vi "Exponential Test.vi"() -> ()   [LabVIEW 2014]
uses:
  <vilib>/Math Plots/3D Math Plots/3D Scatter/3D Scatter XCtrl/3D Scatter.xctl
  <vilib>/Math Plots/3D Math Plots/3D Scatter/3D Scatter Datatype/Public/Plot Helper (Vector).vi
  <vilib>/Analysis/1siggen.llb/Ramp Pattern by Delta.vi
  Math Utilities.lvlib
  <vilib>/Analysis/NI_AALBase.lvlib
  <vilib>/measure/NI_MABase.lvlib
  <vilib>/Math Plots/3D Math Plots/3D Scatter/3D Scatter Datatype/3D Scatter Datatype.lvclass
panel:
  out "Selected Noise Level":dbl
  in  "noise index":i32
  out "etau'":cluster{dbl[], dbl[]}[](graph)=[{[0.0, 0.05, 0.1, 0.15, 0.2, 0.25, 0.3, 0.35, 0.4, 0.45, 0.5, 0.55, 0.6, 0.65, 0.7, 0.75, 0.8, 0.85, 0.9, 0.95, 1.0, 1.05, 1.1, 1.15, 1.2, 1.25, 1.3, 1.35, 1.4, 1.45, 1.5, 1.55, 1.6, 1.65, 1.7, 1.75, 1.8, 1.85, 1.9, 1.95, 2.0, 2.05, 2.1, 2.15, 2.2, 2.25, 2.3, 2.35, 2.4, 2.45, 2.5, 2.55, 2.6, 2.65, 2.7, 2.75, 2.8, 2.85, 2.9, 2.95, 3.0, 3.05, 3.1, 3.15, 3.2, 3.25, 3.3, 3.35, 3.4, 3.45, 3.5, 3.55, 3.6, 3.65, 3.7, 3.75, 3.8, 3.85, 3.9, 3.95, 4.0, 4.05, 4.1, 4.15, 4.2, 4.25, 4.3, 4.35, 4.4, 4.45, 4.5, 4.55, 4.6, 4.65, 4.7, 4.75, 4.8, 4.85, 4.9, 4.95], [0.960541444934628, 1.0300287046137588, 0.8896412059372913, 0.8809320306793802, 0.7883247330312061, 0.8176833763391205, 0.6447128922258879, 0.6273332809368509, 0.6605682518837364, 0.6670014264280115, 0.583805564940926, 0.675732358744051, 0.4639846933111526, 0.6202542521121932, 0.5597277145279371, 0.5135564243561868, 0.5062733727780937, 0.3613578160271843, 0.4475233678516537, 0.3793968608808492, 0.43724877411342006, 0.3597384315625127, 0.2373620816547545, 0.22453592933762084, 0.29842459974751334, 0.3050071640074105, 0.2359236866011837, 0.24302284161365773, 0.23920428907537397, 0.2700720254736181, 0.1918881215092269, 0.2316375620963971, 0.2698374059004593, 0.10938565371609907, 0.18228368619733432, 0.1995904055680095, 0.10262683454287629, 0.12951323626014882, 0.1883316121198414, 0.051005880662942066, 0.1882658145929273, 0.2253474344702741, 0.1072676376138868, 0.05420331503554107, 0.07073686122149538, 0.19072834912888081, 0.06489404614590896, 0.02340665923857653, 0.080727031502262, 0.053160478621205834, 0.1150566849039812, 0.08647339206694683, 0.17225004999139676, 0.14385515421965545, 0.09476811084635094, 0.08535850566392958, 0.042453337460426295, -0.005111835078437502, 0.1266720101202937, 0.08798857698089546, 0.06448330591172151, 0.012535109492323698, -0.02180050629331399, 0.13921091410606592, -0.00448119475112807, 0.025953771409014427, 0.09196924940378937, 0.1251848736523793, 0.09872337746996236, -0.02796928416987523, -0.0439093646999277, 0.07577564143222511, -0.03469012345164275, 0.1000290582787502, 0.07570130581455305, 0.10981843839037647, 0.030883562880611268, 0.05482327411195698, -0.016277970417741722, 0.0739773731669493, 0.11823230258380474, 0.022378034520468177, 0.015118202748243353, 0.06436576688809863, 0.034369714129696256, -0.07590989562072355, 0.11223730777048424, -0.05352288298618646, 0.059251144916092124, -0.054463595365239675, 0.10903521158421503, 0.07349724843361212, -0.04763649889666532, 0.05840026342982382, -0.06312941047179772, -0.04841695002411584, 0.0871009289199655, -0.08241366972549377, 0.06657825659960447, 0.01870496404000565]}, {[0.0, 0.1, 0.2, 0.3, 0.4, 0.5, 0.6, 0.7, 0.8, 0.9, 1.0, 1.1, 1.2, 1.3, 1.4, 1.5, 1.6, 1.7, 1.8, 1.9, 2.0, 2.1, 2.2, 2.3, 2.4, 2.5, 2.6, 2.7, 2.8, 2.9, 3.0, 3.1, 3.2, 3.3, 3.4, 3.5, 3.6, 3.7, 3.8, 3.9, 4.0, 4.1, 4.2, 4.3, 4.4, 4.5, 4.6, 4.7, 4.8, 4.9], [1.0489118049155677, 0.9828657414468108, 0.7287092685494896, 0.7402604459878791, 0.5870346294794287, 0.586721816909444, 0.45440624030548527, 0.5237279303930864, 0.3972561140761981, 0.33254829917367884, 0.34818621735970484, 0.3989198005547301, 0.34947614865970883, 0.20883760536624074, 0.20965525245589398, 0.26857776347019313, 0.23122560558625996, 0.23874984457269088, 0.15561255360224382, 0.1418318343504817, 0.11626272362059906, 0.16392580193843515, 0.033834333279495796, 0.0778706880250746, -0.007929789367372514, 0.005419938340864641, 0.04836411782582296, 0.12887685022889384, 0.15987281329989583, 0.002826123372845442, 0.044361005460079386, 0.01107762227846102, 0.027130325332161268, -0.0329011607483985, -0.00976715691082395, -0.01851382955827155, -0.02912386416561294, 0.05216385233514075, -0.01890067181650635, -0.06324219670124576, -0.06851294508129749, -0.002777132357630538, -0.014512361417010615, 0.08683899542703284, 0.08258002031887463, -0.024344103284262092, 0.0437718075673618, -0.06155030056137617, 0.06644365751447188, 0.05045892575985402]}, {[0.0, 0.2, 0.4, 0.6, 0.8, 1.0, 1.2, 1.4, 1.6, 1.8, 2.0, 2.2, 2.4, 2.6, 2.8, 3.0, 3.2, 3.4, 3.6, 3.8, 4.0, 4.2, 4.4, 4.6, 4.8], [1.0166445888668472, 0.8965127205564365, 0.6746646020918559, 0.5979355379266843, 0.4854152133224972, 0.3872720439703156, 0.3657660253817956, 0.30351089738058307, 0.2198216708301479, 0.20705366479755255, 0.06903085210606028, 0.16530276730729707, 0.15939586940300982, 0.083518667159258, 0.0640925481270926, 0.06369433525293566, 0.04352509905837727, 0.036281546977637566, 0.043303657543107665, 0.08611682194308087, 0.029590496545093097, -0.01733169050921223, -0.024397551503856203, -0.05234666017391198, -0.03711380387257694]}, {[0.0, 0.5, 1.0, 1.5, 2.0, 2.5, 3.0, 3.5, 4.0, 4.5], [1.0623034361710997, 0.5317673867138099, 0.42771698929286195, 0.17661929472640508, 0.05033997654512429, 0.03973823954012479, 0.09664850852882598, 0.07924682307796599, 0.11213514888422532, 0.10083456799625037]}, {[0.0, 1.0, 2.0, 3.0, 4.0], [1.097092230716005, 0.32607780199041114, 0.13609726715261378, 0.0013463089040823967, 0.0574822313090591]}]
  out "tau'":cluster{dbl[], dbl[]}[](graph)=[{[0.0, 0.05, 0.1, 0.15, 0.2, 0.25, 0.3, 0.35, 0.4, 0.45, 0.5, 0.55, 0.6, 0.65, 0.7, 0.75, 0.8, 0.85, 0.9, 0.95, 1.0, 1.05, 1.1, 1.15, 1.2, 1.25, 1.3, 1.35, 1.4, 1.45, 1.5, 1.55, 1.6, 1.65, 1.7, 1.75, 1.8, 1.85, 1.9, 1.95, 2.0, 2.05, 2.1, 2.15, 2.2, 2.25, 2.3, 2.35, 2.4, 2.45, 2.5, 2.55, 2.6, 2.65, 2.7, 2.75, 2.8, 2.85, 2.9, 2.95, 3.0, 3.05, 3.1, 3.15, 3.2, 3.25, 3.3, 3.35, 3.4, 3.45, 3.5, 3.55, 3.6, 3.65, 3.7, 3.75, 3.8, 3.85, 3.9, 3.95, 4.0, 4.05, 4.1, 4.15, 4.2, 4.25, 4.3, 4.35, 4.4, 4.45, 4.5, 4.55, 4.6, 4.65, 4.7, 4.75, 4.8, 4.85, 4.9, 4.95], [0.960541444934628, 1.0300287046137588, 0.8896412059372913, 0.8809320306793802, 0.7883247330312061, 0.8176833763391205, 0.6447128922258879, 0.6273332809368509, 0.6605682518837364, 0.6670014264280115, 0.583805564940926, 0.675732358744051, 0.4639846933111526, 0.6202542521121932, 0.5597277145279371, 0.5135564243561868, 0.5062733727780937, 0.3613578160271843, 0.4475233678516537, 0.3793968608808492, 0.43724877411342006, 0.3597384315625127, 0.2373620816547545, 0.22453592933762084, 0.29842459974751334, 0.3050071640074105, 0.2359236866011837, 0.24302284161365773, 0.23920428907537397, 0.2700720254736181, 0.1918881215092269, 0.2316375620963971, 0.2698374059004593, 0.10938565371609907, 0.18228368619733432, 0.1995904055680095, 0.10262683454287629, 0.12951323626014882, 0.1883316121198414, 0.051005880662942066, 0.1882658145929273, 0.2253474344702741, 0.1072676376138868, 0.05420331503554107, 0.07073686122149538, 0.19072834912888081, 0.06489404614590896, 0.02340665923857653, 0.080727031502262, 0.053160478621205834, 0.1150566849039812, 0.08647339206694683, 0.17225004999139676, 0.14385515421965545, 0.09476811084635094, 0.08535850566392958, 0.042453337460426295, -0.005111835078437502, 0.1266720101202937, 0.08798857698089546, 0.06448330591172151, 0.012535109492323698, -0.02180050629331399, 0.13921091410606592, -0.00448119475112807, 0.025953771409014427, 0.09196924940378937, 0.1251848736523793, 0.09872337746996236, -0.02796928416987523, -0.0439093646999277, 0.07577564143222511, -0.03469012345164275, 0.1000290582787502, 0.07570130581455305, 0.10981843839037647, 0.030883562880611268, 0.05482327411195698, -0.016277970417741722, 0.0739773731669493, 0.11823230258380474, 0.022378034520468177, 0.015118202748243353, 0.06436576688809863, 0.034369714129696256, -0.07590989562072355, 0.11223730777048424, -0.05352288298618646, 0.059251144916092124, -0.054463595365239675, 0.10903521158421503, 0.07349724843361212, -0.04763649889666532, 0.05840026342982382, -0.06312941047179772, -0.04841695002411584, 0.0871009289199655, -0.08241366972549377, 0.06657825659960447, 0.01870496404000565]}, {[0.0, 0.1, 0.2, 0.3, 0.4, 0.5, 0.6, 0.7, 0.8, 0.9, 1.0, 1.1, 1.2, 1.3, 1.4, 1.5, 1.6, 1.7, 1.8, 1.9, 2.0, 2.1, 2.2, 2.3, 2.4, 2.5, 2.6, 2.7, 2.8, 2.9, 3.0, 3.1, 3.2, 3.3, 3.4, 3.5, 3.6, 3.7, 3.8, 3.9, 4.0, 4.1, 4.2, 4.3, 4.4, 4.5, 4.6, 4.7, 4.8, 4.9], [1.0489118049155677, 0.9828657414468108, 0.7287092685494896, 0.7402604459878791, 0.5870346294794287, 0.586721816909444, 0.45440624030548527, 0.5237279303930864, 0.3972561140761981, 0.33254829917367884, 0.34818621735970484, 0.3989198005547301, 0.34947614865970883, 0.20883760536624074, 0.20965525245589398, 0.26857776347019313, 0.23122560558625996, 0.23874984457269088, 0.15561255360224382, 0.1418318343504817, 0.11626272362059906, 0.16392580193843515, 0.033834333279495796, 0.0778706880250746, -0.007929789367372514, 0.005419938340864641, 0.04836411782582296, 0.12887685022889384, 0.15987281329989583, 0.002826123372845442, 0.044361005460079386, 0.01107762227846102, 0.027130325332161268, -0.0329011607483985, -0.00976715691082395, -0.01851382955827155, -0.02912386416561294, 0.05216385233514075, -0.01890067181650635, -0.06324219670124576, -0.06851294508129749, -0.002777132357630538, -0.014512361417010615, 0.08683899542703284, 0.08258002031887463, -0.024344103284262092, 0.0437718075673618, -0.06155030056137617, 0.06644365751447188, 0.05045892575985402]}, {[0.0, 0.2, 0.4, 0.6, 0.8, 1.0, 1.2, 1.4, 1.6, 1.8, 2.0, 2.2, 2.4, 2.6, 2.8, 3.0, 3.2, 3.4, 3.6, 3.8, 4.0, 4.2, 4.4, 4.6, 4.8], [1.0166445888668472, 0.8965127205564365, 0.6746646020918559, 0.5979355379266843, 0.4854152133224972, 0.3872720439703156, 0.3657660253817956, 0.30351089738058307, 0.2198216708301479, 0.20705366479755255, 0.06903085210606028, 0.16530276730729707, 0.15939586940300982, 0.083518667159258, 0.0640925481270926, 0.06369433525293566, 0.04352509905837727, 0.036281546977637566, 0.043303657543107665, 0.08611682194308087, 0.029590496545093097, -0.01733169050921223, -0.024397551503856203, -0.05234666017391198, -0.03711380387257694]}, {[0.0, 0.5, 1.0, 1.5, 2.0, 2.5, 3.0, 3.5, 4.0, 4.5], [1.0623034361710997, 0.5317673867138099, 0.42771698929286195, 0.17661929472640508, 0.05033997654512429, 0.03973823954012479, 0.09664850852882598, 0.07924682307796599, 0.11213514888422532, 0.10083456799625037]}, {[0.0, 1.0, 2.0, 3.0, 4.0], [1.097092230716005, 0.32607780199041114, 0.13609726715261378, 0.0013463089040823967, 0.0574822313090591]}]
  out "output array":dbl[](array[numeric])
  out "Array 3":dbl[](array[numeric])
  out "Array 2":dbl[](array[numeric])
  in  "tau index":i32
  out "3D Scatter":refnum<class "3D Plot Datatype.lvclass">[](xcontrol)
  out "Array":T1(array[cluster])
  in  "taus (us)":dbl[](array[numeric])=[0.5, 1.0, 2.0, 5.0, 10.0, 20.0, 50.0, 100.0, 150.0]
  in  "Noise Levels":dbl[](array[numeric])=[0.0, 0.01, 0.05, 0.1, 0.2, 0.3, 0.4, 0.5, 1.0]
  in  "# Taus":dbl=5.0
  in  "Number of Samples":dbl=4000.0
  out "Taus":T2(graph)=[{"Sampling Frequencies (MHz)"=[20.0, 10.0, 5.0, 2.0, 1.0], [0.9656086307823587, 0.9866685202887719, 1.1569644501410312, 0.7662051282812012, 0.8285928880796682]}, {"Sampling Frequencies (MHz)"=[20.0, 10.0, 5.0, 2.0, 1.0], [0.026104009183676023, 0.034896410998791996, 0.03328061139393245, 0.07782595805221088, 0.07635392209771198]}, {"Sampling Frequencies (MHz)"=[20.0, 10.0, 5.0, 2.0, 1.0], [0.9408079235146063, 0.9408079235146063, 0.9408079235146063, 0.9408079235146063, 0.9408079235146063]}]
  out "Exponential":cluster{dbl[], dbl[]}[](graph)=[{[0.0, 0.05, 0.1, 0.15, 0.2, 0.25, 0.3, 0.35, 0.4, 0.45, 0.5, 0.55, 0.6, 0.65, 0.7, 0.75, 0.8, 0.85, 0.9, 0.95, 1.0, 1.05, 1.1, 1.15, 1.2, 1.25, 1.3, 1.35, 1.4, 1.45, 1.5, 1.55, 1.6, 1.65, 1.7, 1.75, 1.8, 1.85, 1.9, 1.95, 2.0, 2.05, 2.1, 2.15, 2.2, 2.25, 2.3, 2.35, 2.4, 2.45, 2.5, 2.55, 2.6, 2.65, 2.7, 2.75, 2.8, 2.85, 2.9, 2.95, 3.0, 3.05, 3.1, 3.15, 3.2, 3.25, 3.3, 3.35, 3.4, 3.45, 3.5, 3.55, 3.6, 3.65, 3.7, 3.75, 3.8, 3.85, 3.9, 3.95, 4.0, 4.05, 4.1, 4.15, 4.2, 4.25, 4.3, 4.35, 4.4, 4.45, 4.5, 4.55, 4.6, 4.65, 4.7, 4.75, 4.8, 4.85, 4.9, 4.95], [0.960541444934628, 1.0300287046137588, 0.8896412059372913, 0.8809320306793802, 0.7883247330312061, 0.8176833763391205, 0.6447128922258879, 0.6273332809368509, 0.6605682518837364, 0.6670014264280115, 0.583805564940926, 0.675732358744051, 0.4639846933111526, 0.6202542521121932, 0.5597277145279371, 0.5135564243561868, 0.5062733727780937, 0.3613578160271843, 0.4475233678516537, 0.3793968608808492, 0.43724877411342006, 0.3597384315625127, 0.2373620816547545, 0.22453592933762084, 0.29842459974751334, 0.3050071640074105, 0.2359236866011837, 0.24302284161365773, 0.23920428907537397, 0.2700720254736181, 0.1918881215092269, 0.2316375620963971, 0.2698374059004593, 0.10938565371609907, 0.18228368619733432, 0.1995904055680095, 0.10262683454287629, 0.12951323626014882, 0.1883316121198414, 0.051005880662942066, 0.1882658145929273, 0.2253474344702741, 0.1072676376138868, 0.05420331503554107, 0.07073686122149538, 0.19072834912888081, 0.06489404614590896, 0.02340665923857653, 0.080727031502262, 0.053160478621205834, 0.1150566849039812, 0.08647339206694683, 0.17225004999139676, 0.14385515421965545, 0.09476811084635094, 0.08535850566392958, 0.042453337460426295, -0.005111835078437502, 0.1266720101202937, 0.08798857698089546, 0.06448330591172151, 0.012535109492323698, -0.02180050629331399, 0.13921091410606592, -0.00448119475112807, 0.025953771409014427, 0.09196924940378937, 0.1251848736523793, 0.09872337746996236, -0.02796928416987523, -0.0439093646999277, 0.07577564143222511, -0.03469012345164275, 0.1000290582787502, 0.07570130581455305, 0.10981843839037647, 0.030883562880611268, 0.05482327411195698, -0.016277970417741722, 0.0739773731669493, 0.11823230258380474, 0.022378034520468177, 0.015118202748243353, 0.06436576688809863, 0.034369714129696256, -0.07590989562072355, 0.11223730777048424, -0.05352288298618646, 0.059251144916092124, -0.054463595365239675, 0.10903521158421503, 0.07349724843361212, -0.04763649889666532, 0.05840026342982382, -0.06312941047179772, -0.04841695002411584, 0.0871009289199655, -0.08241366972549377, 0.06657825659960447, 0.01870496404000565]}, {[0.0, 0.1, 0.2, 0.3, 0.4, 0.5, 0.6, 0.7, 0.8, 0.9, 1.0, 1.1, 1.2, 1.3, 1.4, 1.5, 1.6, 1.7, 1.8, 1.9, 2.0, 2.1, 2.2, 2.3, 2.4, 2.5, 2.6, 2.7, 2.8, 2.9, 3.0, 3.1, 3.2, 3.3, 3.4, 3.5, 3.6, 3.7, 3.8, 3.9, 4.0, 4.1, 4.2, 4.3, 4.4, 4.5, 4.6, 4.7, 4.8, 4.9], [1.0489118049155677, 0.9828657414468108, 0.7287092685494896, 0.7402604459878791, 0.5870346294794287, 0.586721816909444, 0.45440624030548527, 0.5237279303930864, 0.3972561140761981, 0.33254829917367884, 0.34818621735970484, 0.3989198005547301, 0.34947614865970883, 0.20883760536624074, 0.20965525245589398, 0.26857776347019313, 0.23122560558625996, 0.23874984457269088, 0.15561255360224382, 0.1418318343504817, 0.11626272362059906, 0.16392580193843515, 0.033834333279495796, 0.0778706880250746, -0.007929789367372514, 0.005419938340864641, 0.04836411782582296, 0.12887685022889384, 0.15987281329989583, 0.002826123372845442, 0.044361005460079386, 0.01107762227846102, 0.027130325332161268, -0.0329011607483985, -0.00976715691082395, -0.01851382955827155, -0.02912386416561294, 0.05216385233514075, -0.01890067181650635, -0.06324219670124576, -0.06851294508129749, -0.002777132357630538, -0.014512361417010615, 0.08683899542703284, 0.08258002031887463, -0.024344103284262092, 0.0437718075673618, -0.06155030056137617, 0.06644365751447188, 0.05045892575985402]}, {[0.0, 0.2, 0.4, 0.6, 0.8, 1.0, 1.2, 1.4, 1.6, 1.8, 2.0, 2.2, 2.4, 2.6, 2.8, 3.0, 3.2, 3.4, 3.6, 3.8, 4.0, 4.2, 4.4, 4.6, 4.8], [1.0166445888668472, 0.8965127205564365, 0.6746646020918559, 0.5979355379266843, 0.4854152133224972, 0.3872720439703156, 0.3657660253817956, 0.30351089738058307, 0.2198216708301479, 0.20705366479755255, 0.06903085210606028, 0.16530276730729707, 0.15939586940300982, 0.083518667159258, 0.0640925481270926, 0.06369433525293566, 0.04352509905837727, 0.036281546977637566, 0.043303657543107665, 0.08611682194308087, 0.029590496545093097, -0.01733169050921223, -0.024397551503856203, -0.05234666017391198, -0.03711380387257694]}, {[0.0, 0.5, 1.0, 1.5, 2.0, 2.5, 3.0, 3.5, 4.0, 4.5], [1.0623034361710997, 0.5317673867138099, 0.42771698929286195, 0.17661929472640508, 0.05033997654512429, 0.03973823954012479, 0.09664850852882598, 0.07924682307796599, 0.11213514888422532, 0.10083456799625037]}, {[0.0, 1.0, 2.0, 3.0, 4.0], [1.097092230716005, 0.32607780199041114, 0.13609726715261378, 0.0013463089040823967, 0.0574822313090591]}]
  in  "Run Calc":bool=TRUE
  in  "B":dbl
  in  "A":dbl=1.0
  in  "Sampling Frequencies (MHz)":dbl[](array[numeric])=[20.0, 15.0, 10.0, 8.0, 6.0, 5.0, 2.5, 1.0]
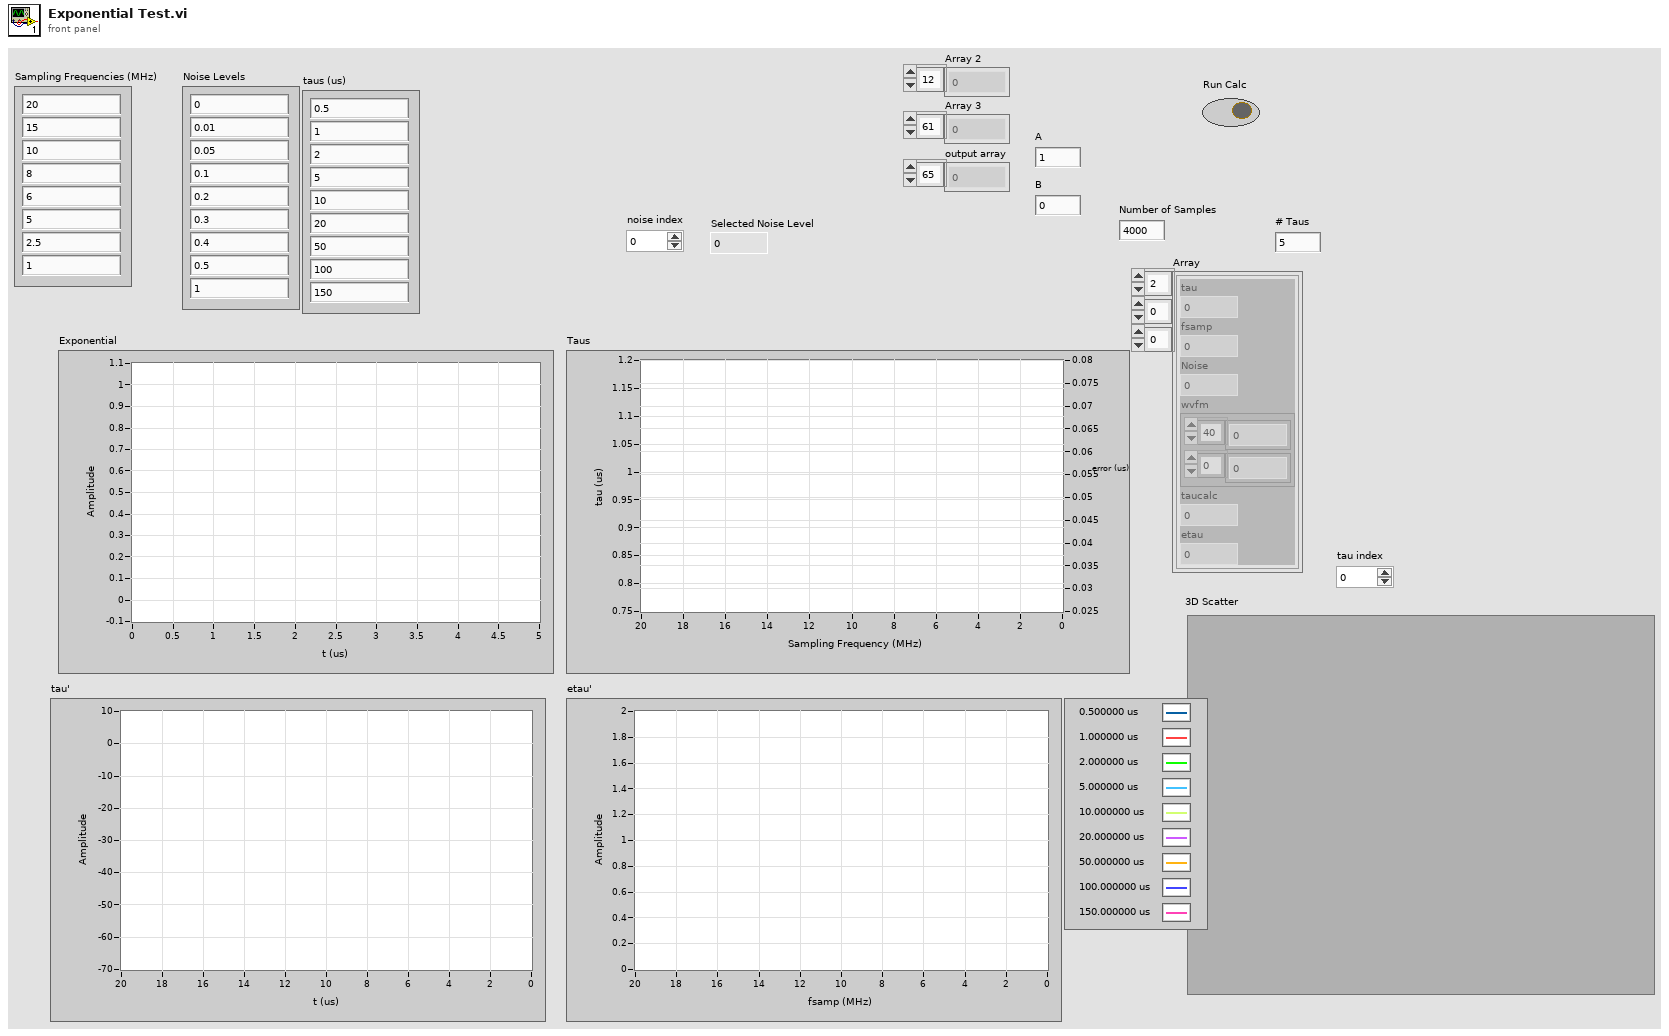
[diagram p1: front panel]
types:
  T1 = cluster{"tau":dbl, "fsamp":dbl, "Noise":dbl, "wvfm":cluster{dbl[], dbl[]}, "taucalc":dbl, "etau":dbl}[][][]
  T2 = cluster{"Sampling Frequencies (MHz)":dbl[], dbl[]}[]
  T3 = cluster{"tau":dbl, "fsamp":dbl, "Noise":dbl, "wvfm":cluster{dbl[], dbl[]}, "taucalc":dbl, "etau":dbl}
  T4 = cluster{dbl, dbl, "Numeric":dbl, cluster{dbl[], dbl[]}, "tau":dbl, "e_tau":dbl}[][][]
  T5 = cluster{"tau":dbl, "fsamp":dbl, "Noise":dbl, "wvfm":cluster{dbl[], dbl[]}, "taucalc":dbl, "etau":dbl}[][]
  T6 = cluster{"tau":dbl, "fsamp":dbl, "Noise":dbl, "wvfm":cluster{dbl[], dbl[]}, "taucalc":dbl, "etau":dbl}[]
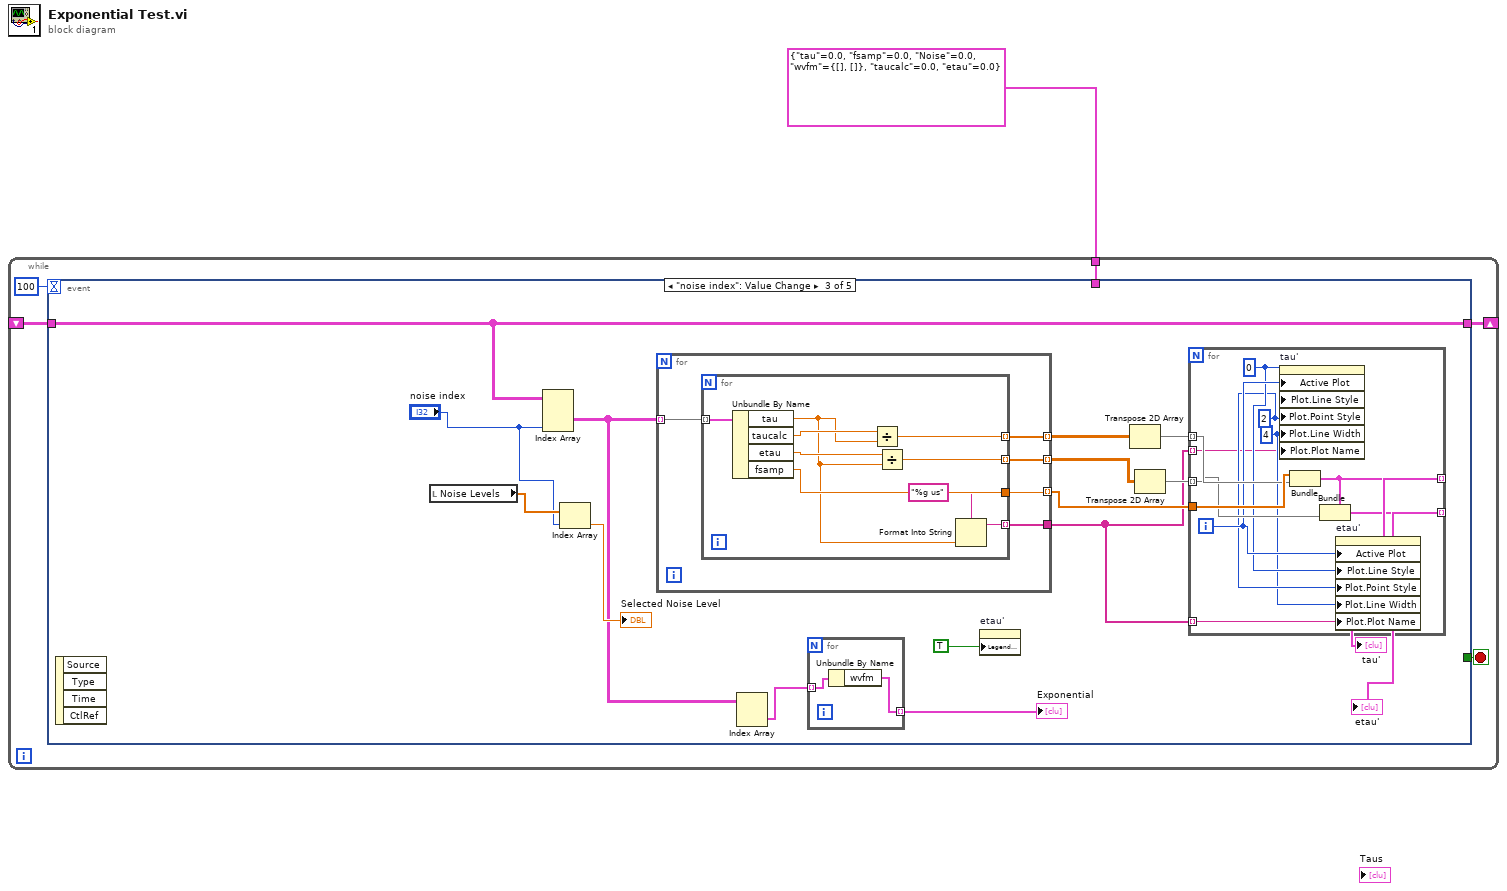
[diagram p0: block diagram]
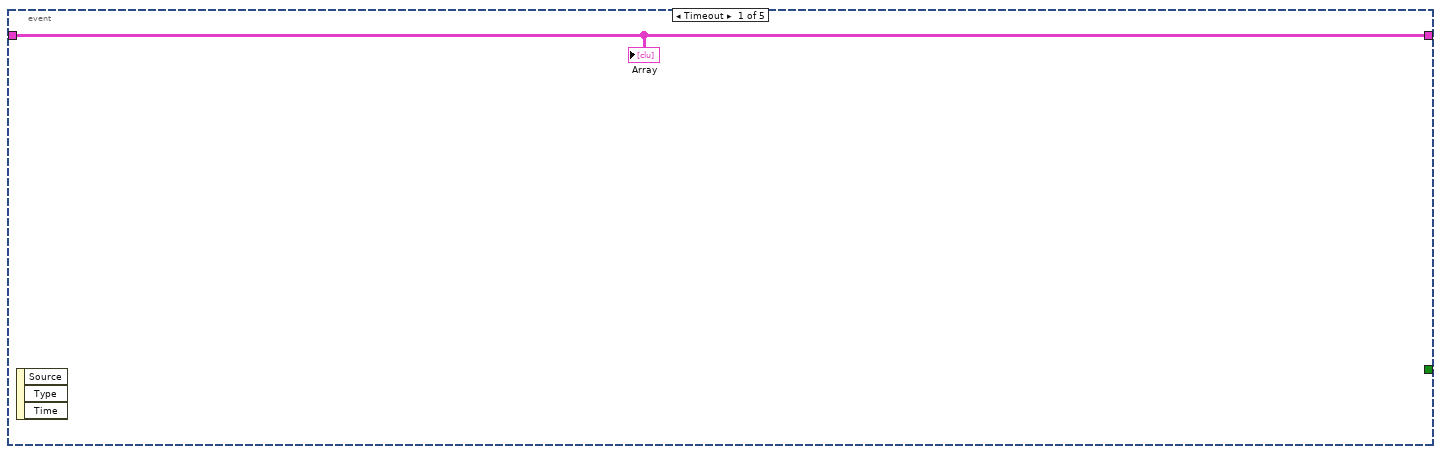
[diagram p2: hidden frame]
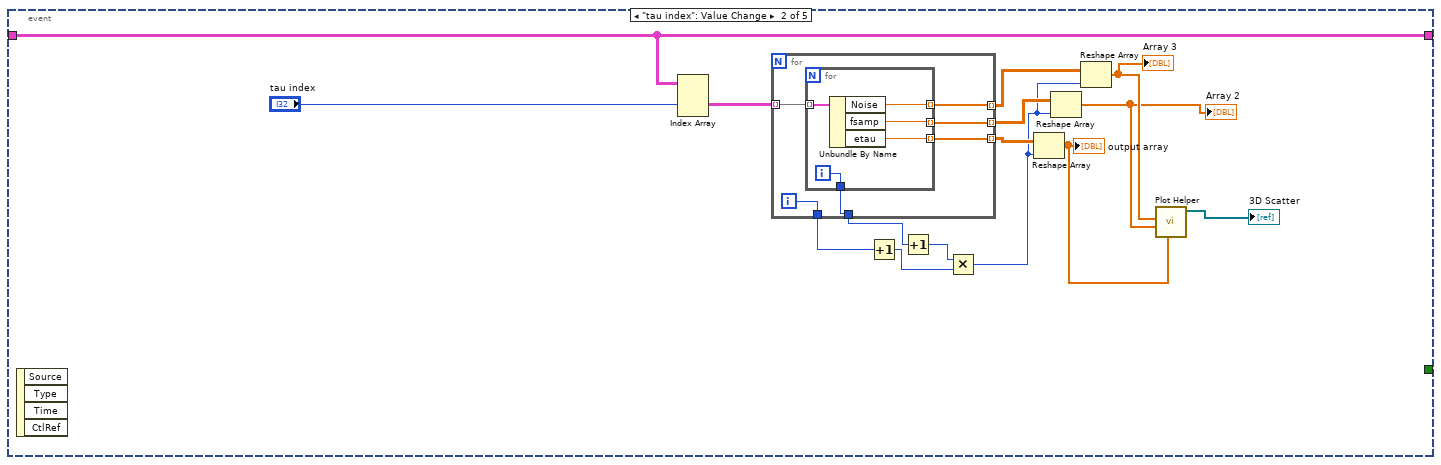
[diagram p3: hidden frame]
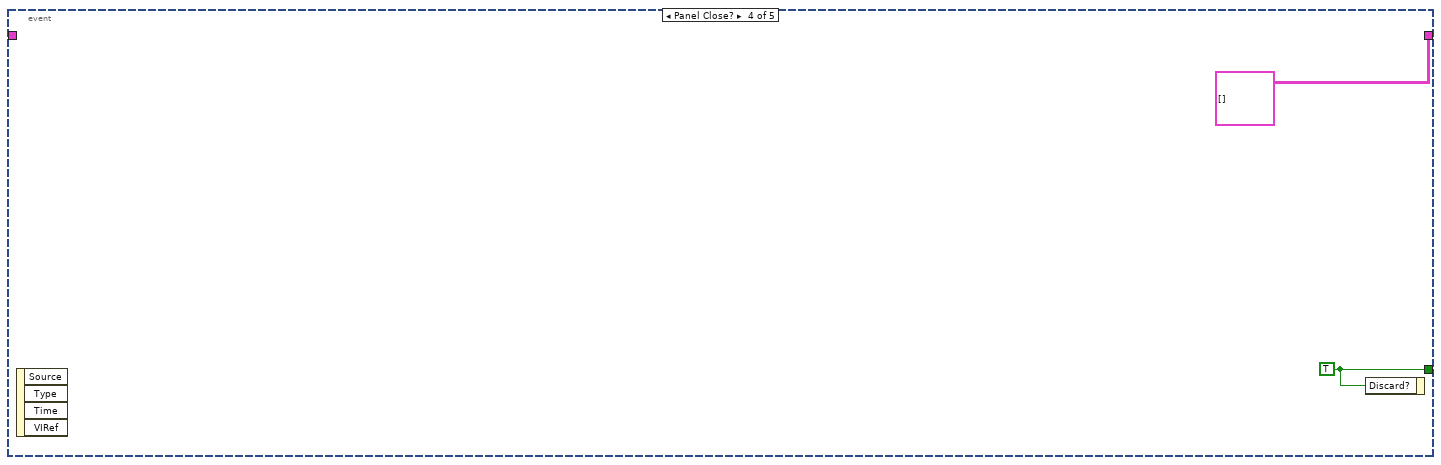
[diagram p4: hidden frame]
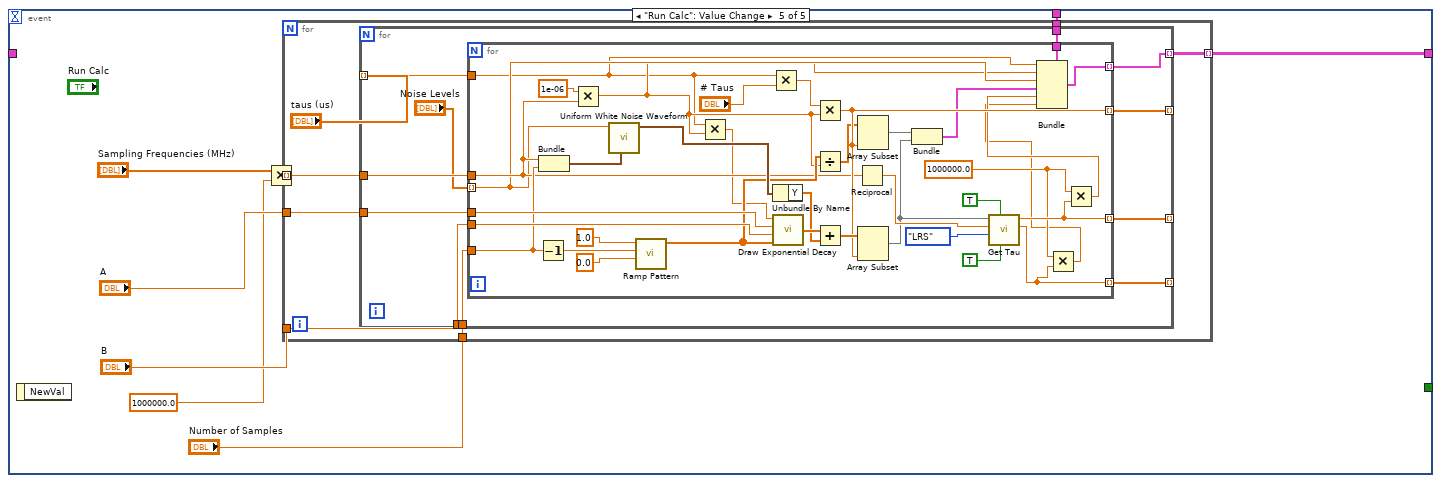
[diagram p5: hidden frame]
diagram:
  n1 = while {
    shift-right: [w5] -> _
    shift-left: _ -> [w4]
    tunnel: T3 {"tau"=0.0, "fsamp"=0.0, "Noise"=0.0, "wvfm"={[], []}, "taucalc"=0.0, "etau"=0.0} ("cluster") -> [w2]
    stop <- w6 stop-if-true
    n2 = event shown="[2] \"noise index\": Value Change" {
      selector: _ -> [_ _ _ _ _]
      dyn-events: _ -> [_ _ _ _ _]
      timeout: 100 -> [_ _ _ _ _]
      tunnel: [_ _ _ w78 _] -> w6
      tunnel: [w7 w22 w49 T4 [] w80] -> w5
      tunnel: w4 -> [w7 w22 w49 _ _]
      tunnel: w2 -> [_ _ _ _ w79]
      event Timeout {
        n3 = event-data() -> ()  [unwired: 1 in, 3 out]
        "Array" <- w7
      }
      event "tau index": Value Change {
        n4 = event-data() -> ()  [unwired: 1 in, 4 out]
        n5 = Index Array(array=w22, index (dim 1)="tau index") -> (element=w21:T5)  [unwired: 2 in]
        n6 = for {
          tunnel: w21 -> [w28] mode=indexing
          tunnel: [w27] -> w15 mode=indexing
          tunnel: [w26] -> w13 mode=indexing
          tunnel: [w25] -> w20 mode=indexing
          tunnel: [w24] -> w18
          tunnel: [w23] -> w19
          i -> [w23]
          n7 = for {
            tunnel: w28 -> [w33] mode=indexing
            tunnel: [w32] -> w26 mode=indexing
            tunnel: [w31] -> w27 mode=indexing
            tunnel: [w30] -> w25 mode=indexing
            tunnel: [w29] -> w24
            i -> [w29]
            n8 = Unbundle By Name(w33) -> ("Noise"=w32:dbl, "fsamp"=w31:dbl, "etau"=w30:dbl)
          }
        }
        n9 = Increment(x=w19) -> (x+1=w16:i32)
        n10 = Increment(x=w18) -> (x+1=w17:i32)
        n11 = Multiply(x=w17, y=w16) -> (x*y=w14:i32)
        n12 = Reshape Array(w20, w14) -> (w11:dbl[])
        "output array" <- w11
        n13 = Reshape Array(w15, w14) -> (w9:dbl[])
        "Array 2" <- w9
        n14 = Reshape Array(w13, w14) -> (w10:dbl[])
        "Array 3" <- w10
        n15 = call-poly <vilib>:"Plot Helper.vi"("z vector"=w11, "y vector"=w9, "x vector"=w10) -> ("3D Plot lvclass Array out"=→"3D Scatter":refnum<class "3D Plot Datatype.lvclass">[])  [unwired: 3 in, 5 out]
      }
      event "noise index": Value Change {
        n16 = event-data() -> ()  [unwired: 1 in, 4 out]
        n17 = local read "Noise Levels"() -> (w39:dbl[])
        n18 = Index Array(array=w49, index (dim 2)="noise index") -> (element=w36:T5)  [unwired: 2 in]
        n19 = Index Array(array=w39, index="noise index") -> (element=→"Selected Noise Level":dbl)
        n20 = for {
          tunnel: w36 -> [w67] mode=indexing
          tunnel: [w66] -> w48 mode=indexing
          tunnel: [w65] -> w47 mode=indexing
          tunnel: [w64] -> w44 mode=indexing
          tunnel: [w63] -> w40
          n21 = for {
            tunnel: w67 -> [w76] mode=indexing
            tunnel: [w71] -> w66 mode=indexing
            tunnel: [w73] -> w65 mode=indexing
            tunnel: [w72] -> w64
            tunnel: [w69] -> w63 mode=indexing
            n22 = Unbundle By Name(w76) -> ("tau"=w68:dbl, "taucalc"=w75:dbl, "etau"=w74:dbl, "fsamp"=w72:dbl)
            n23 = Divide(x=w75, y=w68) -> (x/y=w71:dbl)
            n24 = Divide(x=w74, y=w68) -> (x/y=w73:dbl)
            n25 = Format Into String(format string="%g us", w68) -> (resulting string=w69:string)  [unwired: 2 in, 1 out]
          }
        }
        n26 = Index Array(array=w36) -> (element=w35:T6)  [unwired: 2 in]
        n27 = for {
          tunnel: w35 -> [w51] mode=indexing
          tunnel: [w50] -> w34 mode=indexing
          n28 = Unbundle By Name(w51) -> ("wvfm"=w50:cluster{dbl[], dbl[]})
        }
        "Exponential" <- w34
        n29 = property on="etau'" class="XYGraph (strict)"("Legend Visible"=TRUE ("Legend:Visible")) -> ()  [unwired: 2 in, 2 out]
        n30 = Transpose 2D Array(2D array=w48) -> (transposed array=w46:dbl[][])
        n31 = Transpose 2D Array(2D array=w47) -> (transposed array=w45:dbl[][])
        n32 = for {
          tunnel: w46 -> [w61] mode=indexing
          tunnel: w45 -> [w60] mode=indexing
          tunnel: w44 -> [w62]
          tunnel: [w59] -> w42 mode=indexing
          tunnel: [w58] -> w43 mode=indexing
          tunnel: w40 -> [w53] mode=indexing
          tunnel: w40 -> [w52] mode=indexing
          i -> [w57]
          w54 = u8 4 ("Plot.Line Width")
          w55 = u8 2 ("Plot.Point Style")
          w56 = u8 0 ("Plot.Line Style")
          n33 = property on="tau'" class="XYGraph (strict)"("Active Plot"=w57, "Plot.Line Style"=w56, "Plot.Point Style"=w55, "Plot.Line Width"=w54, "Plot.Plot Name"=w53) -> ()  [unwired: 2 in, 2 out]
          n34 = Bundle(w62, w61) -> (w58:cluster{dbl[], dbl[]})  [unwired: 1 in]
          n35 = Bundle(cluster=w58, w60) -> (w59:cluster{dbl[], dbl[]})  [unwired: 1 in]
          n36 = property on="etau'" class="XYGraph (strict)"("Active Plot"=w57, "Plot.Line Style"=w56, "Plot.Point Style"=w55, "Plot.Line Width"=w54, "Plot.Plot Name"=w52) -> ()  [unwired: 2 in, 2 out]
        }
        "tau'" <- w43
        "etau'" <- w42
      }
      event Panel Close? {
        w78 = TRUE ("Discard?")
        n37 = event-data() -> ()  [unwired: 1 in, 4 out]
        n38 = event-data("Discard?"=w78) -> ()  [unwired: 1 in, 1 out]
      }
      event "Run Calc": Value Change {
        n39 = event-data() -> ()  [unwired: 1 in, 1 out]
        n40 = Multiply(x="Sampling Frequencies (MHz)", y=1000000.0 ("Numeric")) -> (x*y=w83:dbl[])
        n41 = for {
          tunnel: "A" -> [w93]
          tunnel: "B" -> [w92]
          tunnel: "Number of Samples" -> [w91]
          tunnel: w83 -> [w90] mode=indexing
          tunnel: [w88] -> w80 mode=indexing
          tunnel: w79 -> [w87]
          n42 = for {
            tunnel: w93 -> [w104]
            tunnel: w92 -> [w103]
            tunnel: w91 -> [w102]
            tunnel: "taus (us)" -> [w101] mode=indexing
            tunnel: w90 -> [w100]
            tunnel: [w99] -> _ mode=indexing
            tunnel: [w98] -> _ mode=indexing
            tunnel: [w97] -> _ mode=indexing
            tunnel: [w95] -> w88 mode=indexing
            tunnel: w87 -> [w94]
            n43 = for {
              tunnel: w104 -> [w138]
              tunnel: w103 -> [w137]
              tunnel: "Noise Levels" -> [w115] mode=indexing
              tunnel: w102 -> [w130]
              tunnel: [w111] -> w99 mode=indexing
              tunnel: [w109] -> w98 mode=indexing
              tunnel: w101 -> [w105]
              tunnel: [w121] -> w97 mode=indexing
              tunnel: w100 -> [w117]
              tunnel: [w112] -> w95 mode=indexing
              tunnel: w94 -> [w106]
              w108 = 1000000.0 ("Numeric")
              n44 = Decrement(x=w130) -> (x-1=w132:dbl)
              n45 = Bundle("Numeric"=w117, "Number of Samples"=w130) -> (w135:cluster{"Numeric":dbl, "Number of Samples":dbl})  [unwired: 1 in]
              n46 = Multiply(x=1e-06, y=w117) -> (x*y=w114:dbl)
              n47 = call <vilib>:"Uniform White Noise Waveform.vi"("sampling info"=w135, "amplitude"=w115) -> ("signal out"=w136:waveform(dbl))  [unwired: 8 in, 1 out]
              n48 = call-poly <vilib>:"Ramp Pattern.vi"("start"=0.0, "end"=w132, "delta"=1.0) -> ("Ramp Pattern"=w129:dbl[])  [unwired: 6 in, 2 out]
              n49 = Multiply(x=w105, y=w114) -> (x*y=w116:dbl)
              n50 = Multiply(x=w105, y="# Taus") -> (x*y=w124:dbl)
              n51 = Unbundle By Name(w136) -> ("Y"=w133:dbl[])
              n52 = call "Draw Exponential Decay.vi"("time"=w129, "B"=w137, "A"=w138, "tau"=w116) -> ("ExponentialOut"=w134:dbl[])
              n53 = Multiply(x=w124, y=w114) -> (x*y=w121:dbl)
              n54 = Divide(x=w129, y=w114) -> (x/y=w120:dbl[])
              n55 = Add(x=w134, y=w133) -> (x+y=w122:dbl[])
              n56 = Reciprocal(x=w117) -> (1/x=w128:dbl)
              n57 = Array Subset(array=w120, length=w121) -> (w119:dbl[])  [unwired: 1 in]
              n58 = Array Subset(array=w122, length=w121) -> (w118:dbl[])  [unwired: 1 in]
              n59 = Bundle(w119, w118) -> (w113:cluster{dbl[], dbl[]})  [unwired: 1 in]
              n60 = call "Get Tau.vi"("ErrorCallOn"=TRUE, "init"=TRUE, "CalType"=enum8{"DFT-1", "DFT-5", "LRS"}."LRS", "Dt"=w128, "X"=w118) -> ("e_tau"=w109:dbl, "tau"=w111:dbl)  [unwired: 3 in, 2 out]
              n61 = Multiply(x=w108, y=w109) -> (x*y=w107:dbl)
              n62 = Multiply(x=w108, y=w111) -> (x*y=w110:dbl)
              n63 = Bundle(cluster=w106, "tau"=w105, "fsamp"=w114, "Noise"=w115, "wvfm"=w113, "taucalc"=w110, "etau"=w107) -> (w112:T3)
            }
          }
        }
      }
    }
  }
